vi "创建txt文件v1.vi"(6 "是否添加时间？":bool=TRUE, 7 "存储路径":path=path "D:/", 8 "文件头（最后一个字符是换行）":string="Current Voltage\nI V\n", 9 "其他说明信息":string="300K_1000Oe", 10 "测试项目":string="IVcurve", 11 "样品名称":string="deviceUnderTest") -> (2 "文件序号":string, 3 "文件路径":path)   [LabVIEW 2020]
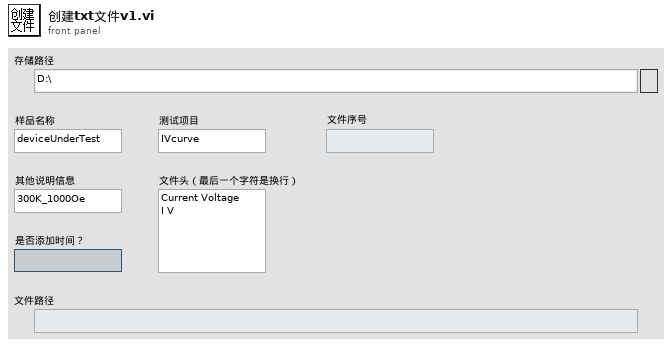
[diagram p1: front panel]
types:
  T1 = enum16{"open", "replace", "create", "open or create", "replace or create", "replace or create with confirmation"}
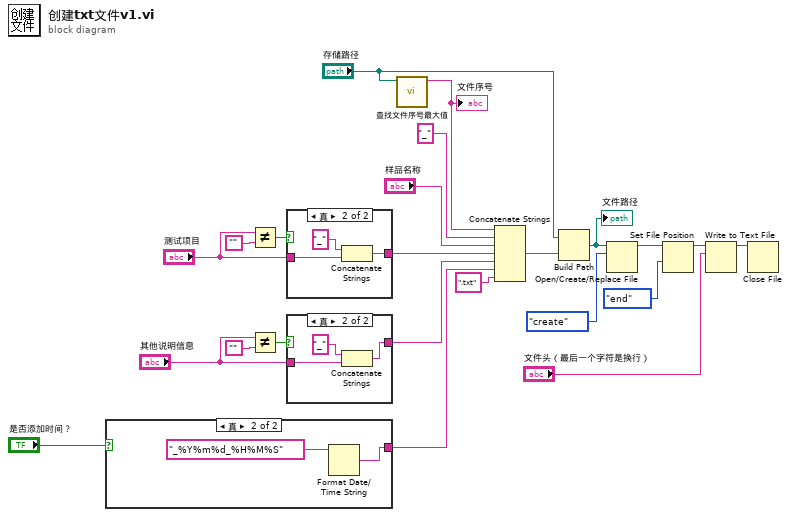
[diagram p0: block diagram]
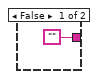
[diagram p2: hidden frame]
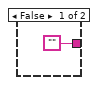
[diagram p3: hidden frame]
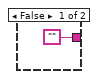
[diagram p4: hidden frame]
diagram:
  n1 = case shown="真" "是否添加时间？" {
    tunnel: ["" w25] -> w13
    frame False {
    }
    frame True {
      n2 = Format Date/Time String(time format string (%c)="_%Y%m%d_%H%M%S" ("时间格式字符串(%c)")) -> (date/time string=w25:string)  [unwired: 2 in]
    }
  }
  n3 = Not Equal?(x="测试项目", y="") -> (x != y?=w21:bool)
  n4 = Not Equal?(x="其他说明信息", y="") -> (x != y?=w18:bool)
  n5 = case shown="真" w21 {
    tunnel: "测试项目" -> [_ w29]
    tunnel: ["" w28] -> w15
    frame False {
    }
    frame True {
      n6 = Concatenate Strings("_" ("字符串"), w29) -> (w28:string)
    }
  }
  n7 = case shown="真" w18 {
    tunnel: "其他说明信息" -> [_ w33]
    tunnel: ["" w32] -> w14
    frame False {
    }
    frame True {
      n8 = Concatenate Strings("_" ("字符串"), w33) -> (w32:string)
    }
  }
  n9 = call "查找文件序号最大值.vi"("存储路径"="存储路径") -> ("文件索引最大值+1"=w2:string)  [unwired: 10 in]
  "文件序号" <- w2
  n10 = Concatenate Strings(w2, "_" ("字符串"), "样品名称", w15, w14, w13, ".txt" ("字符串")) -> (w11:string)
  n11 = Build Path(base path="存储路径", name or relative path=w11) -> (appended path=w5:path)
  "文件路径" <- w5
  n12 = Open/Create/Replace File(file path (use dialog)=w5, operation (0:open)=T1."create" ("操作(0:open)")) -> (refnum out=w10:refnum<file>)  [unwired: 4 in, 2 out]
  n13 = Set File Position(refnum=w10, from (0:start)=enum16{"start", "end", "current"}."end" ("自（0:起始）")) -> (refnum out=w9:refnum<file>)  [unwired: 2 in, 1 out]
  n14 = Write to Text File(file (use dialog)=w9, text="文件头（最后一个字符是换行）") -> (refnum out=w8:refnum<file>)  [unwired: 2 in, 2 out]
  n15 = Close File(refnum=w8) -> ()  [unwired: 1 in, 2 out]
